vi "Pre Launch Init.vi"(11 "System Actor in":refnum<class "System Actor.lvclass">) -> (0 "error out":errorcluster, 3 "System Actor out":refnum<class "System Actor.lvclass">)   [LabVIEW 2014, in "Robot Actor Framework.lvlib" / "System Actor.lvlib" / "System Actor.lvclass"]
doc: "(<B>Filename</B>: Actor Framework.lvlib:Actor.lvclass:Pre Launch Init.vi)\n\nDefines behavior that occurs after the Launch Actor method is invoked but before the actor's Actor Core method begins running.\n\nThe Pre Launch Init method is guaranteed to finish before the Launch Actor method returns to its caller and before the actor itself receives any messages. Any references that the Pre Launch Init method obtains are guaranteed to have the same lifetime as the actor itself. Any errors that the Pre Launch Init method returns will abort the launch.\n\nBy default, this method does nothing. A descendant class may override it to define behavior."
uses:
  System Actor.lvclass
  System Actor.lvclass/System Actor.ctl
  <vilib>/ActorFramework/Actor/Actor.lvclass
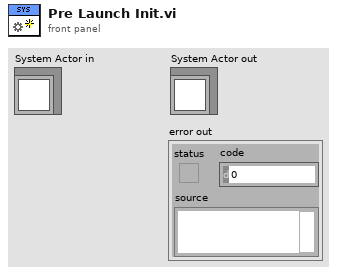
[diagram p1: front panel]
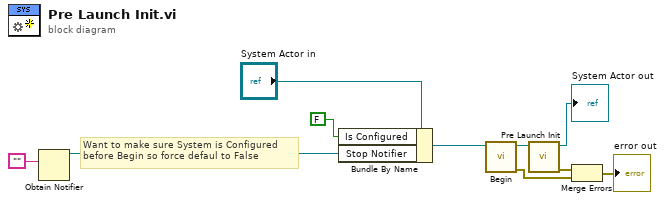
[diagram p0: block diagram]
diagram:
  # "Want to make sure System is Configured\nbefore Begin so force defaul to False"
  n1 = Obtain Notifier(notification data type="") -> (notifier out=w5:refnum<notifier>)  [unwired: 3 in, 2 out]
  n2 = Bundle By Name(cluster="System Actor in", "Is Configured"=FALSE, "Stop Notifier"=w5) -> (w1:refnum<class "System Actor.lvclass">)
  n3 = call-dynamic "Begin.vi"("System Actor in"=w1) -> ("error out"=w2:errorcluster, "System Actor out"=w4:refnum<class "System Actor.lvclass">)  [unwired: 9 in]
  n4 = call-parent "Pre Launch Init.vi"("Actor in"=w4) -> ("error out"=w10:errorcluster, "Actor out"=→"System Actor out":refnum<class "System Actor.lvclass">)  [unwired: 9 in]
  n5 = Merge Errors(w10, w2) -> (→"error out":errorcluster)
